vi "SLSC Initilize Properties.vi"(8 "error in (no error)":errorcluster, 11 "Capabilities":T2={"vendorNum"=0, "vendorName"="", "vendorPrefix"="", "productNum"=0, "productName"="", "capsVersion"="", "capsSpecVersion"=0, "capsSpecOldestCompatibleVersion"=1, "enums"=[], "properties"=[], "commands"=[], "scales"=[], "physicalChannels"=[], "registerMap"={"registers"=[]}}) -> (0 "error out":errorcluster, 1 "productNum":u32, 2 "vendorNum":u32, 3 "Configuration Data":T9={"Properties"={"Boolean Properties"=[], "Double Properties"=[], "I32 Properties"=[], "I64 Properties"=[], "String Properties"=[], "U32 Properties"=[], "U64 Properties"=[]}, "Commands"=[], "Reset Commands"=[], "Apply Values on Deployment"=TRUE, "Apply Reset on Undeployment"=TRUE, "Change Commands"=[]}, 4 "Identification":T1={"vendorName"="", "productNum"=0, "capsVersion"="", "capsSpecVersion"=0, "productName"="", "vendorNum"=0, "vendorPrefix"="", "capsSpecOldestCompatibleVersion"=1})   [LabVIEW 2020, in "SLSC EDS System Explorer.lvlib"]
uses:
  SLSC EDS System Explorer.lvlib
  Shared/SLSC Static Settings.ctl
  SLSC CD API/SLSC CD Engine/SLSC Dynamic Channel.ctl
  SLSC CD API/SLSC CD Engine/SLSC Datatype.ctl
  SLSC EDS API/JSON parsing/physicalChannel.ctl
  SLSC EDS API/JSON parsing/command.ctl
  SLSC EDS API/JSON parsing/property.ctl
  SLSC EDS API/JSON parsing/EDSjsonStructure.ctl
  SLSC EDS API/JSON parsing/enum.ctl
  SLSC EDS API/JSON parsing/scale.ctl
  SLSC EDS API/JSON parsing/register.ctl
  SLSC CD API/SLSC CD Engine/SLSC Identification.ctl
  Shared/Compiled.Settings
  SLSC CD API/SLSC CD Shared/SLSC CD Shared.lvlib
  Shared/SLSC EDS Shared.lvlib
panel:
  out "Properties to be applied":T7[](array[typedef])
  # "not working\nregisterMap->registers->initialValue"
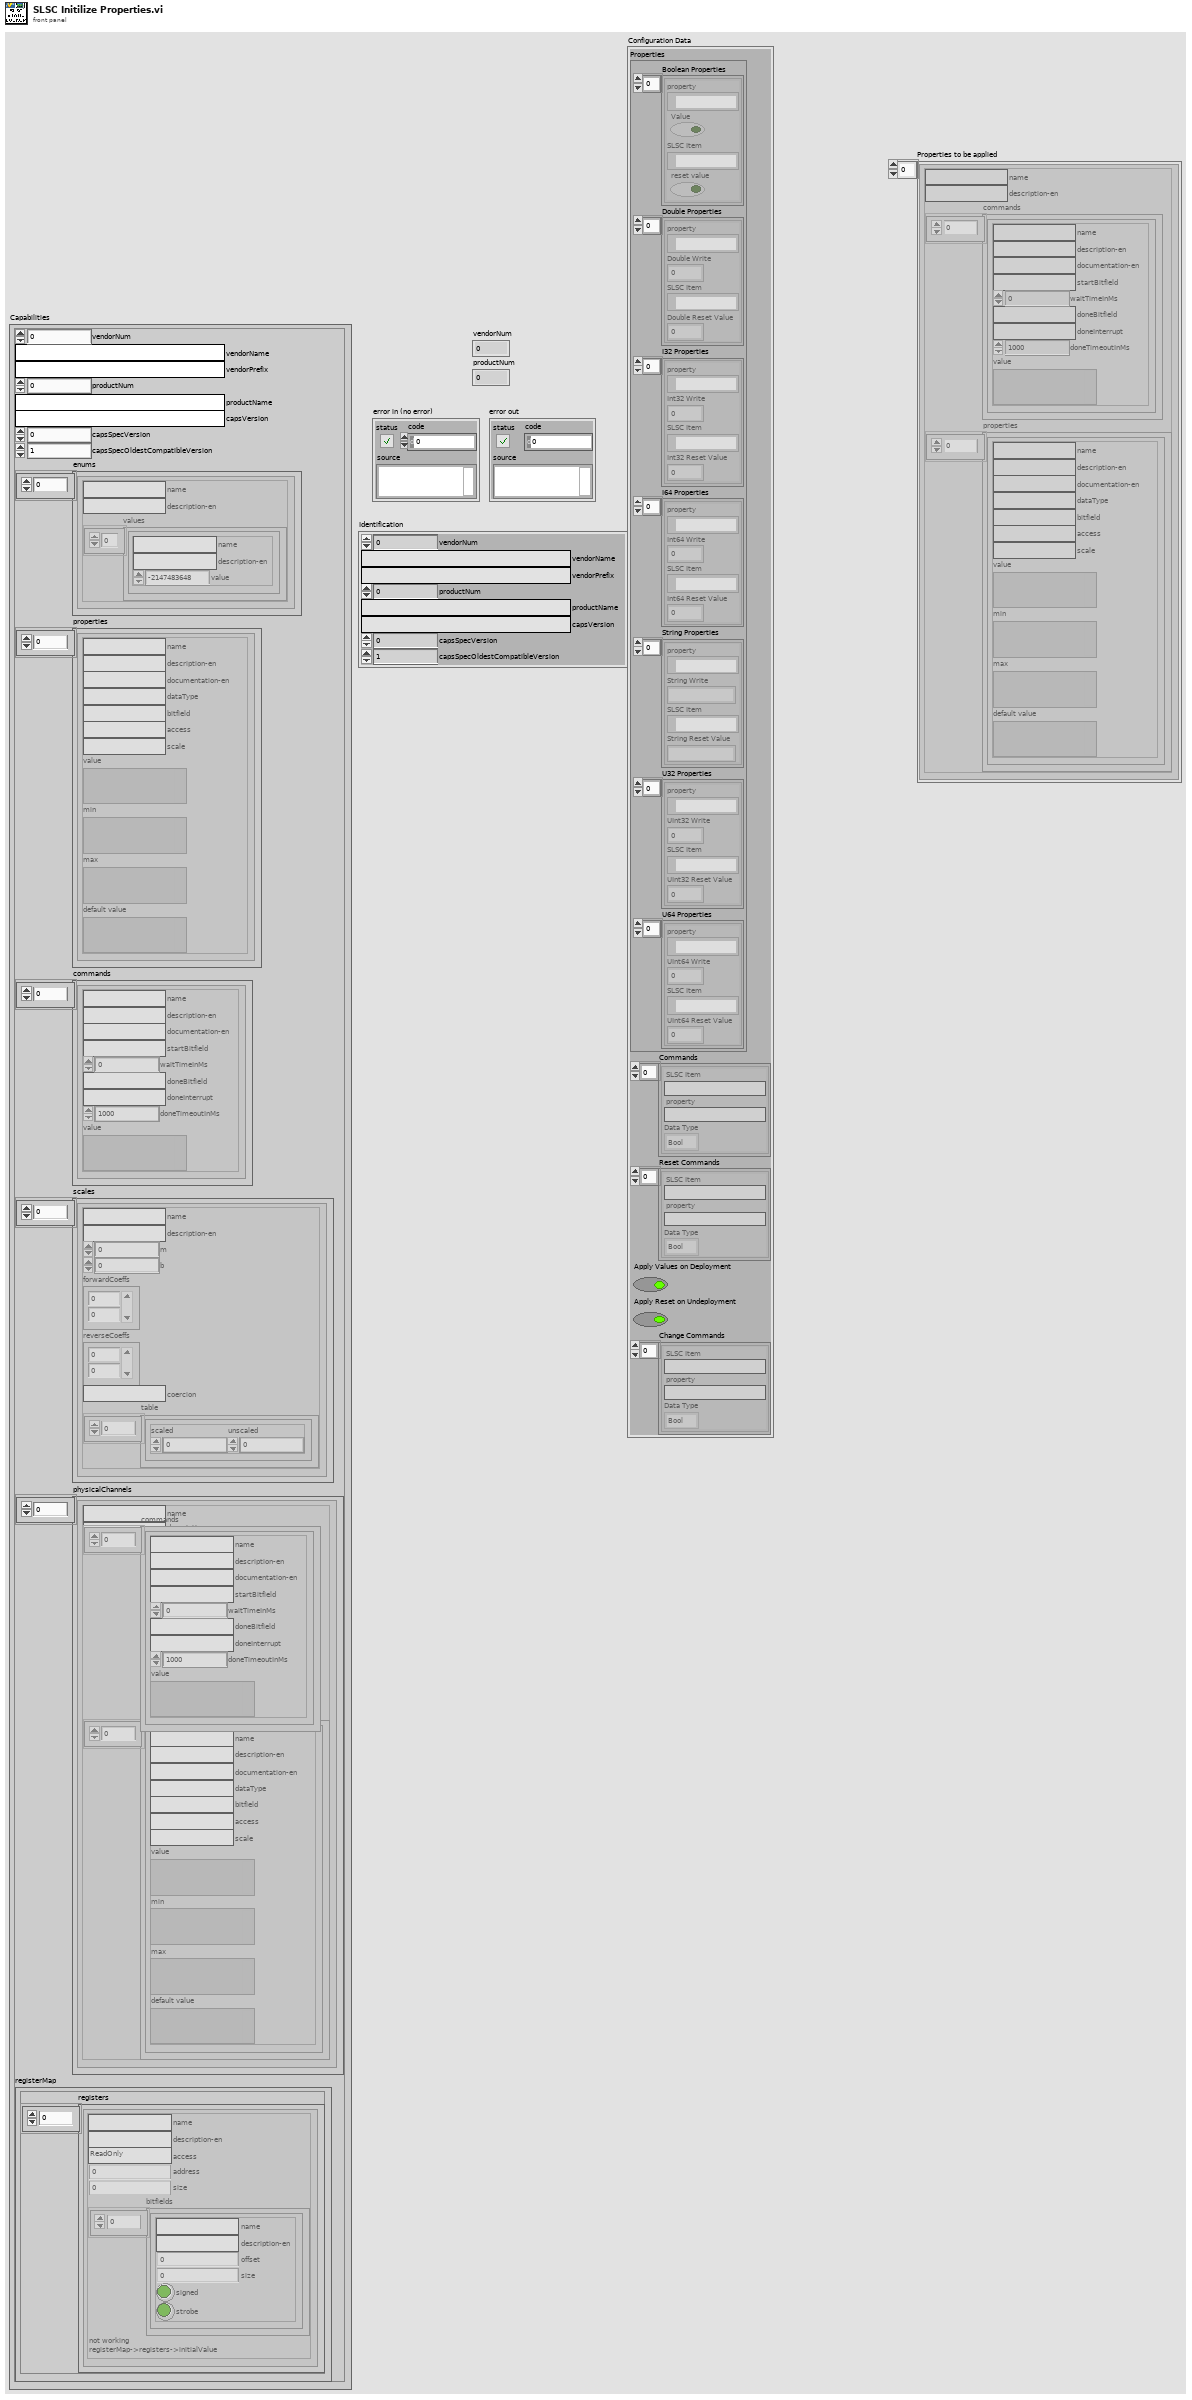
[diagram p1: front panel]
types:
  T1 = typedef "SLSC CD Shared.lvlib/SLSC Identification.ctl" = cluster{"vendorName":string, "productNum":u32, "capsVersion":string, "capsSpecVersion":u32, "productName":string, "vendorNum":u32, "vendorPrefix":string, "capsSpecOldestCompatibleVersion":u32}
  T2 = typedef "EDSjsonStructure.ctl" = cluster{"vendorNum":u32, "vendorName":string, "vendorPrefix":string, "productNum":u32, "productName":string, "capsVersion":string, "capsSpecVersion":u32, "capsSpecOldestCompatibleVersion":u32, "enums":T3[], "properties":T4[], "commands":T5[], "scales":T6[], "physicalChannels":T7[], "registerMap":cluster{"registers":T8[]}}
  T3 = typedef "enum.ctl" = cluster{"name":string, "description-en":string, "values":cluster{"name":string, "description-en":string, "value":i32}[]}
  T4 = typedef "property.ctl" = cluster{"name":string, "description-en":string, "documentation-en":string, "dataType":string, "bitfield":string, "access":string, "scale":string, "value":variant, "min":variant, "max":variant, "default value":variant}
  T5 = typedef "command.ctl" = cluster{"name":string, "description-en":string, "documentation-en":string, "startBitfield":string, "waitTimeInMs":i32, "doneBitfield":string, "doneInterrupt":string, "doneTimeoutInMs":i32, "value":variant}
  T6 = typedef "scale.ctl" = cluster{"name":string, "description-en":string, "m":dbl, "b":dbl, "forwardCoeffs":dbl[], "reverseCoeffs":dbl[], "coercion":string, "table":cluster{"scaled":dbl, "unscaled":dbl}[]}
  T7 = typedef "physicalChannel.ctl" = cluster{"name":string, "description-en":string, "commands":T5[], "properties":T4[]}
  T8 = typedef "register.ctl" = cluster{"name":string, "description-en":string, "access":string, "address":u32, "size":u32, "bitfields":cluster{"name":string, "description-en":string, "offset":u32, "size":u32, "signed":bool, "strobe":bool}[]}
  T9 = typedef "SLSC EDS Shared.lvlib/SLSC Static Settings.ctl" = cluster{"Properties":cluster{"Boolean Properties":cluster{"property":refnum<k21>, "Value":bool, "SLSC Item":refnum<k21>, "reset value":bool}[], "Double Properties":cluster{"property":refnum<k21>, "Double Write":dbl, "SLSC Item":refnum<k21>, "Double Reset Value":dbl}[], "I32 Properties":cluster{"property":refnum<k21>, "Int32 Write":i32, "SLSC Item":refnum<k21>, "Int32 Reset Value":i32}[], "I64 Properties":cluster{"property":refnum<k21>, "Int64 Write":i64, "SLSC Item":refnum<k21>, "Int64 Reset Value":i64}[], "String Properties":cluster{"property":refnum<k21>, "String Write":string, "SLSC Item":refnum<k21>, "String Reset Value":string}[], "U32 Properties":cluster{"property":refnum<k21>, "UInt32 Write":u32, "SLSC Item":refnum<k21>, "UInt32 Reset Value":u32}[], "U64 Properties":cluster{"property":refnum<k21>, "UInt64 Write":u64, "SLSC Item":refnum<k21>, "UInt64 Reset Value":u64}[]}, "Commands":T10[], "Reset Commands":T10[], "Apply Values on Deployment":bool, "Apply Reset on Undeployment":bool, "Change Commands":T10[]}
  T10 = typedef "SLSC CD Shared.lvlib/SLSC Dynamic Channel.ctl" = cluster{"SLSC Item":string, "property":string, "Data Type":T11}
  T11 = typedef "SLSC CD Shared.lvlib/SLSC Datatype.ctl" = enum16{"Bool", "Double", "I32", "I64", "String", "U32", "U64"}
  T12 = typedef "SLSC EDS Shared.lvlib/Compiled.Settings" = cluster{"Name":string, "SLSC Name or IP Address":string, "Slot #":i32, "Configuration Data":T9, "SLSC Get/Read Properties":T10[], "SLSC Set/Write Properties":T10[], "SLSC Dynamic Commands":T10[], "Support Modules":cluster{"Dev.ProductNumber":u32, "Dev.VendorNumber":u32}[]}
  T13 = enum16{"Bool", "Double", "I32", "I64", "String", "U32", "U64"}
  T14 = cluster{"property":refnum<k21>, "Value":bool, "SLSC Item":refnum<k21>, "reset value":bool}[]
  T15 = cluster{"property":refnum<k21>, "Value":bool, "SLSC Item":refnum<k21>, "reset value":bool}
  T16 = cluster{"property":refnum<k21>, "Double Write":dbl, "SLSC Item":refnum<k21>, "Double Reset Value":dbl}[]
  T17 = cluster{"property":refnum<k21>, "Double Write":dbl, "SLSC Item":refnum<k21>, "Double Reset Value":dbl}
  T18 = cluster{"property":refnum<k21>, "Int32 Write":i32, "SLSC Item":refnum<k21>, "Int32 Reset Value":i32}[]
  T19 = cluster{"property":refnum<k21>, "Int32 Write":i32, "SLSC Item":refnum<k21>, "Int32 Reset Value":i32}
  T20 = cluster{"property":refnum<k21>, "Int64 Write":i64, "SLSC Item":refnum<k21>, "Int64 Reset Value":i64}[]
  T21 = cluster{"property":refnum<k21>, "Int64 Write":i64, "SLSC Item":refnum<k21>, "Int64 Reset Value":i64}
  T22 = cluster{"property":refnum<k21>, "String Write":string, "SLSC Item":refnum<k21>, "String Reset Value":string}[]
  T23 = cluster{"property":refnum<k21>, "String Write":string, "SLSC Item":refnum<k21>, "String Reset Value":string}
  T24 = cluster{"property":refnum<k21>, "UInt32 Write":u32, "SLSC Item":refnum<k21>, "UInt32 Reset Value":u32}[]
  T25 = cluster{"property":refnum<k21>, "UInt32 Write":u32, "SLSC Item":refnum<k21>, "UInt32 Reset Value":u32}
  T26 = cluster{"property":refnum<k21>, "UInt64 Write":u64, "SLSC Item":refnum<k21>, "UInt64 Reset Value":u64}[]
  T27 = cluster{"property":refnum<k21>, "UInt64 Write":u64, "SLSC Item":refnum<k21>, "UInt64 Reset Value":u64}
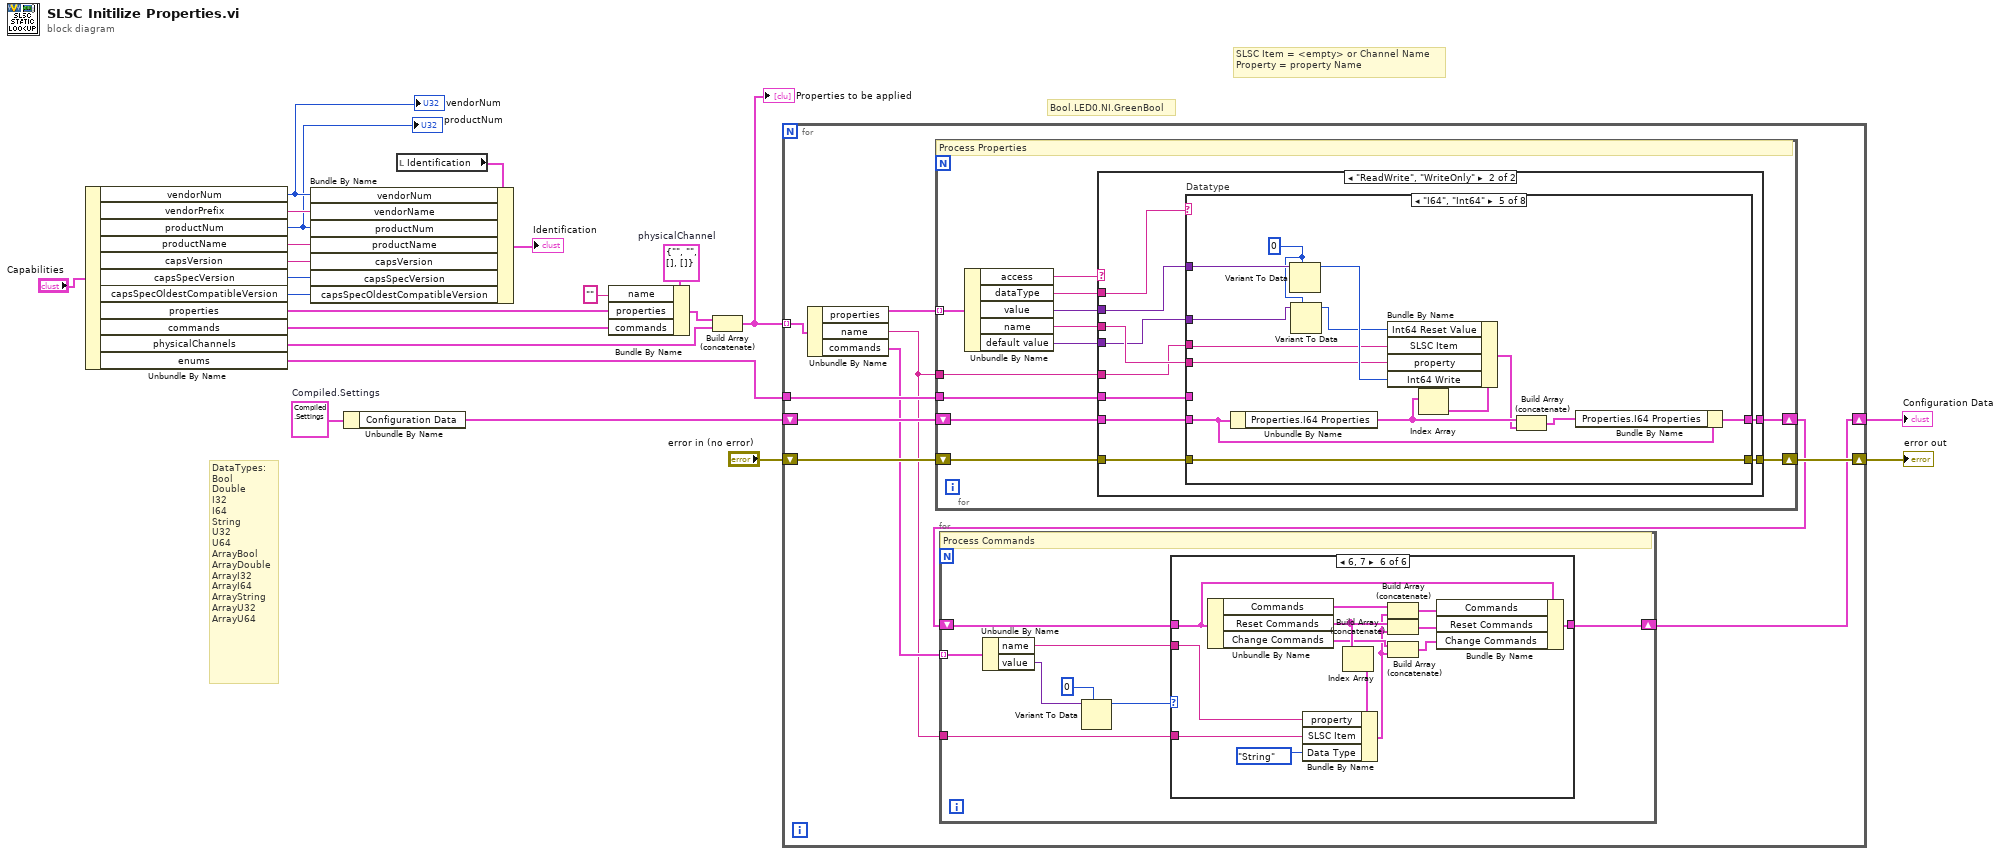
[diagram p0: block diagram]
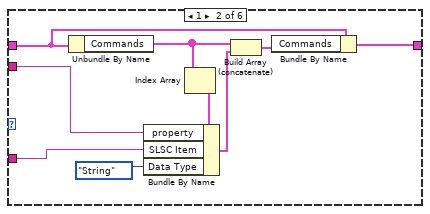
[diagram p3: hidden frame]
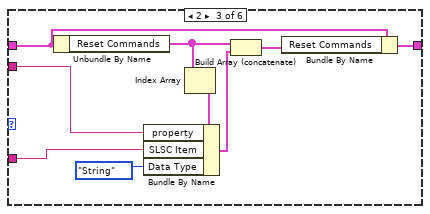
[diagram p4: hidden frame]
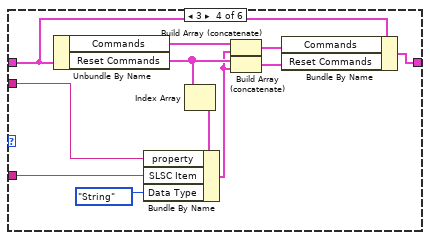
[diagram p5: hidden frame]
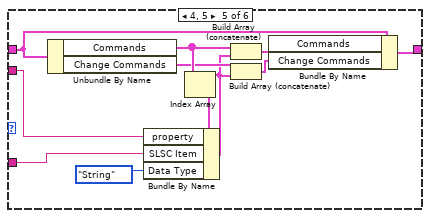
[diagram p6: hidden frame]
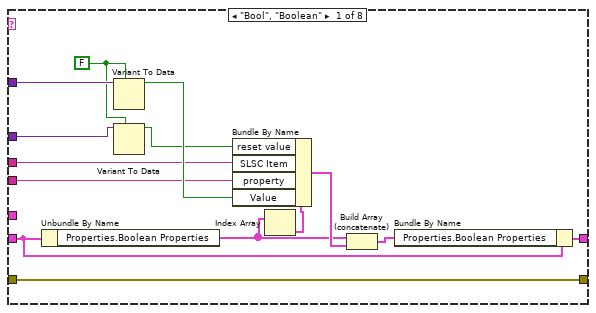
[diagram p8: hidden frame]
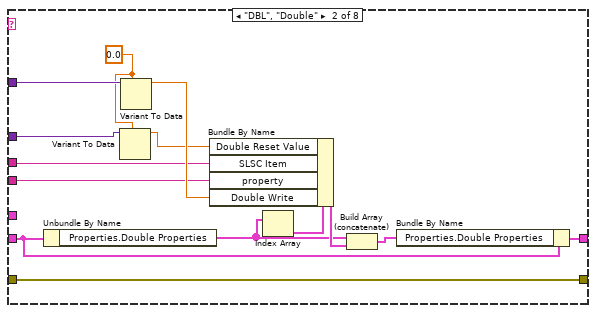
[diagram p9: hidden frame]
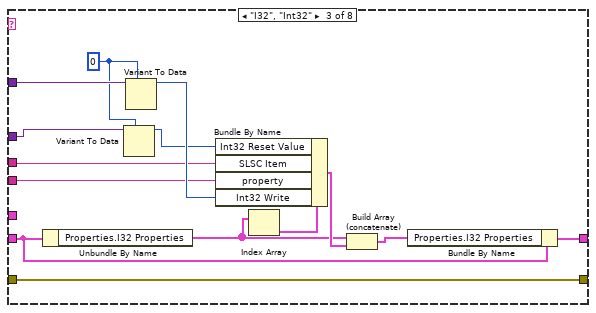
[diagram p10: hidden frame]
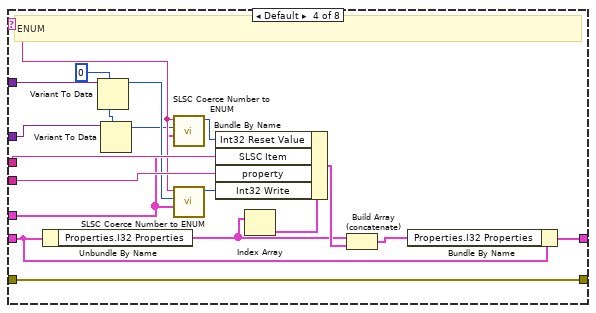
[diagram p11: hidden frame]
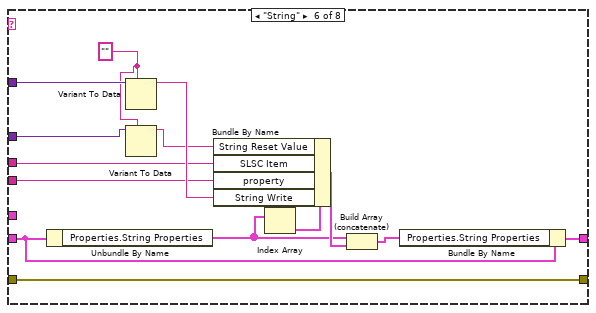
[diagram p12: hidden frame]
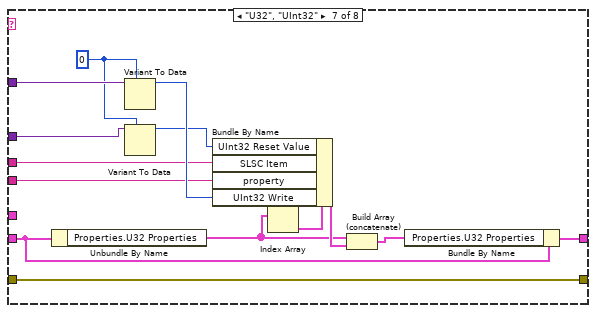
[diagram p13: hidden frame]
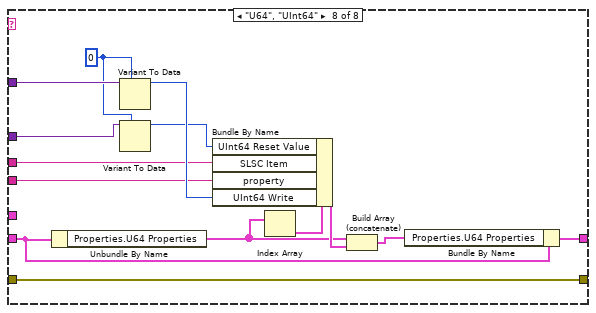
[diagram p14: hidden frame]
diagram:
  w18 = T7 {"name"="", "description-en"="", "commands"=[], "properties"=[]}  # physicalChannel
  w21 = T12 {"Name"="", "SLSC Name or IP Address"="", "Slot #"=0, "Configuration Data"={"Properties"={"Boolean Properties"=[], "Double Properties"=[], "I32 Properties"=[], "I64 Properties"=[], "String Properties"=[], "U32 Properties"=[], "U64 Properties"=[]}, "Commands"=[], "Reset Commands"=[], "Apply Values on Deployment"=TRUE, "Apply Reset on Undeployment"=TRUE, "Change Commands"=[]}, "SLSC Get/Read Properties"=[], "SLSC Set/Write Properties"=[], "SLSC Dynamic Commands"=[], "Support Modules"=[]}  # Compiled.Settings
  # "SLSC Item = <empty> or Channel Name\nProperty = property Name"
  # "DataTypes:\nBool\nDouble\nI32\nI64\nString\nU32\nU64\nArrayBool\nArrayDouble\nArrayI32\nArrayI64\nArrayString\nArrayU32\nArrayU64"
  # "Bool.LED0.NI.GreenBool"
  n1 = Unbundle By Name("Capabilities") -> ("vendorNum"=w2:u32, "vendorPrefix"=w6:string, "productNum"=w1:u32, "productName"=w5:string, "capsVersion"=w4:string, "capsSpecVersion"=w3:u32, "capsSpecOldestCompatibleVersion"=w7:u32, "properties"=w16:T4[], "commands"=w12:T5[], "physicalChannels"=w11:T7[], "enums"=w10:T3[])
  "vendorNum" <- w2
  "productNum" <- w1
  n2 = Unbundle By Name(w21) -> ("Configuration Data"=w20:T9)
  n3 = local read "Identification"() -> (w9:T1)
  n4 = Bundle By Name(cluster=w9, "vendorNum"=w2, "vendorName"=w6, "productNum"=w1, "productName"=w5, "capsVersion"=w4, "capsSpecVersion"=w3, "capsSpecOldestCompatibleVersion"=w7) -> (→"Identification":T1)
  n5 = Bundle By Name(cluster=w18, "name"="", "properties"=w16, "commands"=w12) -> (w15:T7)
  n6 = Build Array (concatenate)(w15, w11) -> (w19:T7[])
  "Properties to be applied" <- w19
  n7 = for {
    shift-right: [w25] -> w23
    shift-left: w20 -> [w32]
    shift-right: [w33] -> w22
    shift-left: "error in (no error)" -> [w31]
    tunnel: w19 -> [w30] mode=indexing
    tunnel: w10 -> [w28]
    n8 = Unbundle By Name(w30) -> ("properties"=w29:T4[], "name"=w24:string, "commands"=w27:T5[])
    n9 = for {
      shift-right: [w105] -> w33
      shift-left: w31 -> [w100]
      shift-right: [w107] -> w26
      shift-left: w32 -> [w106]
      tunnel: w29 -> [w104] mode=indexing
      tunnel: w24 -> [w99]
      tunnel: w28 -> [w98]
      # "Process Properties"
      n10 = Unbundle By Name(w104) -> ("access"=w97:string, "dataType"=w103:string, "value"=w102:variant, "name"=w101:string, "default value"=w96:variant)
      n11 = case shown="\"ReadWrite\", \"WriteOnly\"" w97 {
        tunnel: [w108 w119] -> w107
        tunnel: w106 -> [w108 w118]
        tunnel: [w109 w117] -> w105
        tunnel: w103 -> [_ w116]
        tunnel: w102 -> [_ w115]
        tunnel: w101 -> [_ w114]
        tunnel: w100 -> [w109 w113]
        tunnel: w99 -> [_ w112]
        tunnel: w98 -> [_ w111]
        tunnel: w96 -> [_ w110]
        frame Default {
        }
        frame "ReadWrite", "WriteOnly" {
          n12 = case "Datatype" shown="\"I64\", \"Int64\"" w116 {
            selector: w116 -> [_ _ _ w167 _ _ _ _]
            tunnel: w113 -> [w120 w134 w148 w162 w180 w194 w208 w222]
            tunnel: w118 -> [w128 w146 w156 w175 w189 w202 w216 w230]
            tunnel: [w131 w144 w159 w177 w192 w205 w219 w233] -> w119
            tunnel: [w120 w134 w148 w162 w180 w194 w208 w222] -> w117
            tunnel: w115 -> [w130 w142 w157 w176 w190 w203 w217 w231]
            tunnel: w114 -> [w127 w140 w154 w173 w187 w200 w214 w228]
            tunnel: w112 -> [w126 w141 w155 w174 w188 w201 w215 w229]
            tunnel: w111 -> [_ _ _ w166 _ _ _ _]
            tunnel: w110 -> [w122 w136 w150 w164 w182 w196 w209 w223]
            frame "Bool", "Boolean" {
              w123 = FALSE
              n13 = Unbundle By Name(w128) -> ("Properties.Boolean Properties"=w125:T14)
              n14 = Variant To Data(type=w123, Variant=w130) -> (data=w129:bool)  [unwired: 1 in, 1 out]
              n15 = Variant To Data(type=w123, Variant=w122) -> (data=w121:bool)  [unwired: 1 in, 1 out]
              n16 = Index Array(array=w125) -> (element=w124:T15)  [unwired: 1 in]
              n17 = Bundle By Name(cluster=w124, "reset value"=w121, "SLSC Item"=w126, "property"=w127, "Value"=w129) -> (w133:T15)
              n18 = Build Array (concatenate)(w125, w133) -> (w132:T14)
              n19 = Bundle By Name(cluster=w128, "Properties.Boolean Properties"=w132) -> (w131:T9)
            }
            frame "DBL", "Double" {
              w137 = 0.0
              n20 = Unbundle By Name(w146) -> ("Properties.Double Properties"=w139:T16)
              n21 = Variant To Data(type=w137, Variant=w136) -> (data=w135:dbl)  [unwired: 1 in, 1 out]
              n22 = Variant To Data(type=w137, Variant=w142) -> (data=w143:dbl)  [unwired: 1 in, 1 out]
              n23 = Index Array(array=w139) -> (element=w138:T17)  [unwired: 1 in]
              n24 = Bundle By Name(cluster=w138, "Double Reset Value"=w135, "SLSC Item"=w141, "property"=w140, "Double Write"=w143) -> (w147:T17)
              n25 = Build Array (concatenate)(w139, w147) -> (w145:T16)
              n26 = Bundle By Name(cluster=w146, "Properties.Double Properties"=w145) -> (w144:T9)
            }
            frame "I32", "Int32" {
              w151 = 0
              n27 = Unbundle By Name(w156) -> ("Properties.I32 Properties"=w153:T18)
              n28 = Variant To Data(type=w151, Variant=w150) -> (data=w149:i32)  [unwired: 1 in, 1 out]
              n29 = Variant To Data(type=w151, Variant=w157) -> (data=w158:i32)  [unwired: 1 in, 1 out]
              n30 = Index Array(array=w153) -> (element=w152:T19)  [unwired: 1 in]
              n31 = Bundle By Name(cluster=w152, "Int32 Reset Value"=w149, "SLSC Item"=w155, "property"=w154, "Int32 Write"=w158) -> (w161:T19)
              n32 = Build Array (concatenate)(w153, w161) -> (w160:T18)
              n33 = Bundle By Name(cluster=w156, "Properties.I32 Properties"=w160) -> (w159:T9)
            }
            frame Default {
              w165 = 0
              # "ENUM"
              n34 = Unbundle By Name(w175) -> ("Properties.I32 Properties"=w170:T18)
              n35 = Variant To Data(type=w165, Variant=w176) -> (data=w171:i32)  [unwired: 1 in, 1 out]
              n36 = Variant To Data(type=w165, Variant=w164) -> (data=w163:i32)  [unwired: 1 in, 1 out]
              n37 = call "SLSC Coerce Number to ENUM.vi"("enums"=w166, "Enum in"=w163, "dataType"=w167) -> ("Enum out"=w168:i32)  [unwired: 7 in, 1 out]
              n38 = call "SLSC Coerce Number to ENUM.vi"("enums"=w166, "Enum in"=w171, "dataType"=w167) -> ("Enum out"=w172:i32)  [unwired: 7 in, 1 out]
              n39 = Index Array(array=w170) -> (element=w169:T19)  [unwired: 1 in]
              n40 = Bundle By Name(cluster=w169, "Int32 Reset Value"=w168, "SLSC Item"=w174, "property"=w173, "Int32 Write"=w172) -> (w179:T19)
              n41 = Build Array (concatenate)(w170, w179) -> (w178:T18)
              n42 = Bundle By Name(cluster=w175, "Properties.I32 Properties"=w178) -> (w177:T9)
            }
            frame "I64", "Int64" {
              w183 = i64 0
              n43 = Unbundle By Name(w189) -> ("Properties.I64 Properties"=w186:T20)
              n44 = Variant To Data(type=w183, Variant=w190) -> (data=w191:i64)  [unwired: 1 in, 1 out]
              n45 = Variant To Data(type=w183, Variant=w182) -> (data=w181:i64)  [unwired: 1 in, 1 out]
              n46 = Index Array(array=w186) -> (element=w185:T21)  [unwired: 1 in]
              n47 = Bundle By Name(cluster=w185, "Int64 Reset Value"=w181, "SLSC Item"=w188, "property"=w187, "Int64 Write"=w191) -> (w184:T21)
              n48 = Build Array (concatenate)(w186, w184) -> (w193:T20)
              n49 = Bundle By Name(cluster=w189, "Properties.I64 Properties"=w193) -> (w192:T9)
            }
            frame "String" {
              w197 = ""
              n50 = Unbundle By Name(w202) -> ("Properties.String Properties"=w199:T22)
              n51 = Variant To Data(type=w197, Variant=w203) -> (data=w204:string)  [unwired: 1 in, 1 out]
              n52 = Variant To Data(type=w197, Variant=w196) -> (data=w195:string)  [unwired: 1 in, 1 out]
              n53 = Index Array(array=w199) -> (element=w198:T23)  [unwired: 1 in]
              n54 = Bundle By Name(cluster=w198, "String Reset Value"=w195, "SLSC Item"=w201, "property"=w200, "String Write"=w204) -> (w207:T23)
              n55 = Build Array (concatenate)(w199, w207) -> (w206:T22)
              n56 = Bundle By Name(cluster=w202, "Properties.String Properties"=w206) -> (w205:T9)
            }
            frame "U32", "UInt32" {
              w213 = u32 0
              n57 = Unbundle By Name(w216) -> ("Properties.U32 Properties"=w212:T24)
              n58 = Variant To Data(type=w213, Variant=w217) -> (data=w218:u32)  [unwired: 1 in, 1 out]
              n59 = Variant To Data(type=w213, Variant=w209) -> (data=w210:u32)  [unwired: 1 in, 1 out]
              n60 = Index Array(array=w212) -> (element=w211:T25)  [unwired: 1 in]
              n61 = Bundle By Name(cluster=w211, "UInt32 Reset Value"=w210, "SLSC Item"=w215, "property"=w214, "UInt32 Write"=w218) -> (w221:T25)
              n62 = Build Array (concatenate)(w212, w221) -> (w220:T24)
              n63 = Bundle By Name(cluster=w216, "Properties.U32 Properties"=w220) -> (w219:T9)
            }
            frame "U64", "UInt64" {
              w227 = u64 0
              n64 = Unbundle By Name(w230) -> ("Properties.U64 Properties"=w226:T26)
              n65 = Variant To Data(type=w227, Variant=w231) -> (data=w232:u64)  [unwired: 1 in, 1 out]
              n66 = Variant To Data(type=w227, Variant=w223) -> (data=w224:u64)  [unwired: 1 in, 1 out]
              n67 = Index Array(array=w226) -> (element=w225:T27)  [unwired: 1 in]
              n68 = Bundle By Name(cluster=w225, "UInt64 Reset Value"=w224, "SLSC Item"=w229, "property"=w228, "UInt64 Write"=w232) -> (w235:T27)
              n69 = Build Array (concatenate)(w226, w235) -> (w234:T26)
              n70 = Bundle By Name(cluster=w230, "Properties.U64 Properties"=w234) -> (w233:T9)
            }
          }
        }
      }
    }
    n71 = for {
      tunnel: w27 -> [w41] mode=indexing
      shift-right: [w36] -> w25
      shift-left: w26 -> [w37]
      tunnel: w24 -> [w34]
      # "Process Commands"
      n72 = Unbundle By Name(w41) -> ("name"=w35:string, "value"=w39:variant)
      n73 = Variant To Data(type=u32 0 ("number"), Variant=w39) -> (data=w38:u32)  [unwired: 1 in, 1 out]
      n74 = case shown="6, 7" w38 {
        tunnel: w37 -> [w42 w51 w60 w71 w82 w95]
        tunnel: [w42 w46 w55 w67 w78 w92] -> w36
        tunnel: w35 -> [_ w44 w53 w65 w76 w90]
        tunnel: w34 -> [_ w43 w52 w64 w75 w89]
        frame 0, Default {
        }
        frame 1 {
          n75 = Unbundle By Name(w51) -> ("Commands"=w48:T10[])
          n76 = Index Array(array=w48) -> (element=w50:T10)  [unwired: 1 in]
          n77 = Bundle By Name(cluster=w50, "property"=w44, "SLSC Item"=w43, "Data Type"=T13."String") -> (w49:T10)
          n78 = Build Array (concatenate)(w48, w49) -> (w47:T10[])
          n79 = Bundle By Name(cluster=w51, "Commands"=w47) -> (w46:T9)
        }
        frame 2 {
          n80 = Unbundle By Name(w60) -> ("Reset Commands"=w57:T10[])
          n81 = Index Array(array=w57) -> (element=w59:T10)  [unwired: 1 in]
          n82 = Bundle By Name(cluster=w59, "property"=w53, "SLSC Item"=w52, "Data Type"=T13."String") -> (w58:T10)
          n83 = Build Array (concatenate)(w57, w58) -> (w56:T10[])
          n84 = Bundle By Name(cluster=w60, "Reset Commands"=w56) -> (w55:T9)
        }
        frame 3 {
          n85 = Unbundle By Name(w71) -> ("Commands"=w63:T10[], "Reset Commands"=w69:T10[])
          n86 = Index Array(array=w69) -> (element=w70:T10)  [unwired: 1 in]
          n87 = Bundle By Name(cluster=w70, "property"=w65, "SLSC Item"=w64, "Data Type"=T13."String") -> (w62:T10)
          n88 = Build Array (concatenate)(w63, w62) -> (w61:T10[])
          n89 = Build Array (concatenate)(w69, w62) -> (w68:T10[])
          n90 = Bundle By Name(cluster=w71, "Commands"=w61, "Reset Commands"=w68) -> (w67:T9)
        }
        frame 4, 5 {
          n91 = Unbundle By Name(w82) -> ("Commands"=w80:T10[], "Change Commands"=w74:T10[])
          n92 = Index Array(array=w80) -> (element=w81:T10)  [unwired: 1 in]
          n93 = Bundle By Name(cluster=w81, "property"=w76, "SLSC Item"=w75, "Data Type"=T13."String") -> (w73:T10)
          n94 = Build Array (concatenate)(w80, w73) -> (w79:T10[])
          n95 = Build Array (concatenate)(w74, w73) -> (w72:T10[])
          n96 = Bundle By Name(cluster=w82, "Commands"=w79, "Change Commands"=w72) -> (w78:T9)
        }
        frame 6, 7 {
          n97 = Unbundle By Name(w95) -> ("Commands"=w88:T10[], "Reset Commands"=w93:T10[], "Change Commands"=w86:T10[])
          n98 = Index Array(array=w93) -> (element=w94:T10)  [unwired: 1 in]
          n99 = Bundle By Name(cluster=w94, "property"=w90, "SLSC Item"=w89, "Data Type"=T13."String") -> (w85:T10)
          n100 = Build Array (concatenate)(w88, w85) -> (w87:T10[])
          n101 = Build Array (concatenate)(w93, w85) -> (w83:T10[])
          n102 = Build Array (concatenate)(w86, w85) -> (w84:T10[])
          n103 = Bundle By Name(cluster=w95, "Commands"=w87, "Reset Commands"=w83, "Change Commands"=w84) -> (w92:T9)
        }
      }
    }
  }
  "Configuration Data" <- w23
  "error out" <- w22
